vi "CRYStimulus Table Insert.vi"(9 "Insert":bool, 10 "Stimulus TableRef":refnum<vi>, 11 "Flatten Stimulus Setup String":string) -> (2 "Stimulus TableRef out":refnum<vi>)   [LabVIEW 2013]
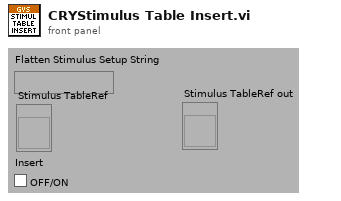
[diagram p1: front panel]
types:
  T1 = typedef "CRYfstepsw.ctl" = cluster{"Level(U)":dbl, "Start Freq(Hz)":dbl, "Stop Freq(Hz)":dbl, "ML val level name":string, "Use ML Val level?":bool, "ML axis":u8, "Steps (#)":i32, "Cycles/step(#)":u32, "Time/step (s)":dbl, "Step Resolution":u16, "unit":u16, "Start Freq Name":string, "Stop Freq Name":string, "Start Freq Axis":u8, "Stop Freq Axis":u8, "Start Freq Flag":string, "Stop Freq Flag":string, "Output Imp":dbl, "Nominal Imp":dbl, "V on DUT":bool}
  T2 = typedef "CRYflogsw.ctl" = cluster{"Level(U)":dbl, "Start Freq(Hz)":dbl, "Stop Freq(Hz)":dbl, "Sweep Rate(s/dec)":dbl, "Use ML Val level?":bool, "ML val level name":string, "ML axis":u8, "TSR params":cluster{"FSamp":dbl, "FStart":dbl, "FStop":dbl, "NOffset":dbl, "MStop":dbl, "MStart":dbl, "NHarm":dbl, "Tsamp":dbl, "Amplit":dbl}, "unit":u16, "Start Freq Name":string, "Stop Freq Name":string, "Start Freq Axis":u8, "Stop Freq Axis":u8, "Start Freq Flag":string, "Stop Freq Flag":string, "Output Imp":dbl, "Nominal Imp":dbl, "V on DUT":bool}
  T3 = typedef "CRYampsw.ctl" = cluster{"Freq(Hz)":dbl, "Steps (#)":i32, "Cycles(#)":u32, "Use ML Val freq?":bool, "ML val freq name":string, "ML axis":u8, "Start Ampl(U)":dbl, "Stop Ampl(U)":dbl, "unit":u16}
  T4 = typedef "CRYwavefile.ctl" = cluster{"Level(U)":dbl, "Wave Path":string, "ML axis":u8, "ML val level name":string, "Use ML Val level?":bool, "wave info":string, "wave time":string, "Peak value4":dbl, "RMS value4":dbl, "wave channel":u16, "unit":u16, "Output Imp":dbl, "Nominal Imp":dbl, "V on DUT":bool}
  T5 = typedef "CRYdcconn.ctl" = cluster{"dc ctrl":u16, "dcmax I":u16, "dc polar":u16, "dc ctrl":u16, "Steps (#)":i32, "Time/step (s)":dbl, "Start Ampl(U)":dbl, "Stop Ampl(U)":dbl, "Level(U)":dbl, "Step Size":dbl}
  T6 = typedef "CRYtwotone.ctl" = cluster{"Steps (#)":i32, "Tone Type":u8, "Freq2(Hz)":dbl, "Time/step (s)":dbl, "Cycles/step (#)":u32, "ML val level name":string, "Use ML Val level?":bool, "Level(U) 2":dbl, "Diff Freq(Hz)":dbl, "ML axis 2":u8, "Diff/Ratio":u8, "Level(U)":dbl, "Stop Freq(Hz)":dbl, "Ratio Val":dbl, "ML val level name 2":string, "Use ML Val level? 2":bool, "ML axis":u8, "Start Freq(Hz)":dbl, "Step Resolution":u16, "Ratio":u16, "TabCtrl6":enum32{"Master Tone", "Slave Tone"}, "unit 1":u16, "unit 2":u16, "Start Freq Name":string, "Stop Freq Name":string, "Start Freq Axis":u8, "Stop Freq Axis":u8, "Start Freq Flag":string, "Stop Freq Flag":string}
  T7 = typedef "CRYmltitone.ctl" = cluster{"Level(U)":dbl, "Min Freq(Hz)":dbl, "Max Freq(Hz)":dbl, "Duration(s)":dbl, "Freq Rounding":bool, "Rounding Val":dbl, "Profile":i32, "ML axis 2":u8, "ML val level name":string, "Use ML Val level?":bool, "ML axis":u8, "Step Resolution":u16, "unit":u16, "Start Freq Name":string, "Stop Freq Name":string, "Start Freq Axis":u8, "Stop Freq Axis":u8, "Start Freq Flag":string, "Stop Freq Flag":string, "Output Imp":dbl, "Nominal Imp":dbl, "V on DUT":bool}
  T8 = typedef "CRYnoise.ctl" = cluster{"Noise Type":u8, "Min Freq(Hz)":dbl, "Max Freq(Hz)":dbl, "Level(U)":dbl, "Duration(s)":dbl, "ML val level name":string, "Use ML Val level?":bool, "ML axis":u8, "unit":u16, "Start Freq Name":string, "Stop Freq Name":string, "Start Freq Axis":u8, "Stop Freq Axis":u8, "Start Freq Flag":string, "Stop Freq Flag":string, "Output Imp":dbl, "Nominal Imp":dbl, "V on DUT":bool}
  T9 = cluster{"fstepsw":T1, "flogsw":T2, "ampsw":T3, "wavefile":T4, "dcconn":T5, "twotone":T6, "mltitone":T7, "noise":T8, "sqwvsw":cluster{"Level(U)":dbl, "Duty Cycle":dbl, "ML val level name":string, "ML axis":u8, "Start Freq(Hz)":u32, "Stop Freq(Hz)":u32, "Use ML Val level?":bool, "Steps (#)":u32, "Cycles/step (#)":u32, "Time/step (s)":dbl, "Step Resolution":u16}, "tnbrst":cluster{"Level(U)":dbl, "ML val level name":string, "ML axis":u8, "Start Freq(Hz)":u32, "Use ML Val level?":bool, "Cycles/step (#)":u32, "Duration(s)":dbl}}
  T10 = cluster{"Data Type":string, "Version":u16, "Dimension":u8}
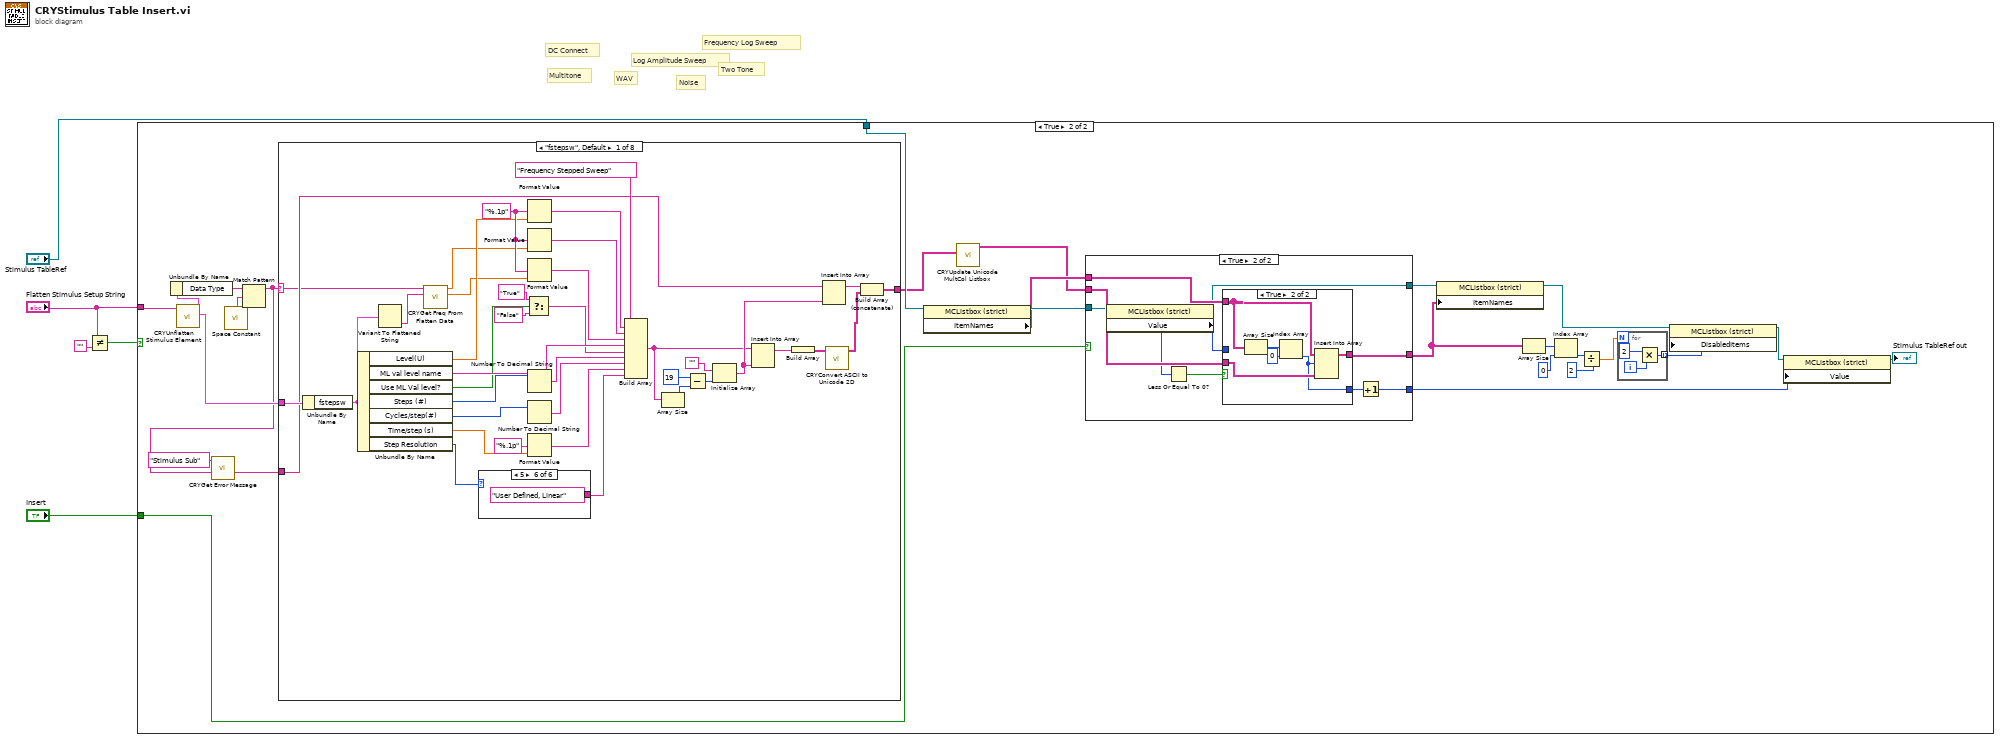
[diagram p0: block diagram]
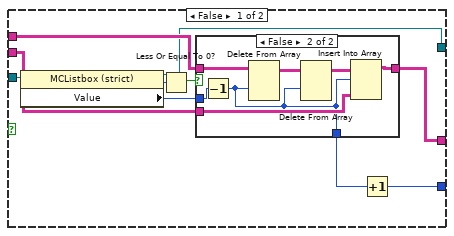
[diagram p3: hidden frame]
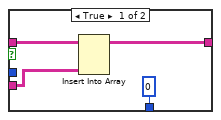
[diagram p4: hidden frame]
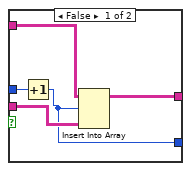
[diagram p5: hidden frame]
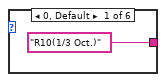
[diagram p6: hidden frame]
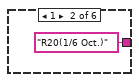
[diagram p7: hidden frame]
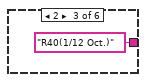
[diagram p8: hidden frame]
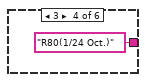
[diagram p9: hidden frame]
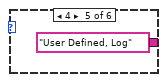
[diagram p10: hidden frame]
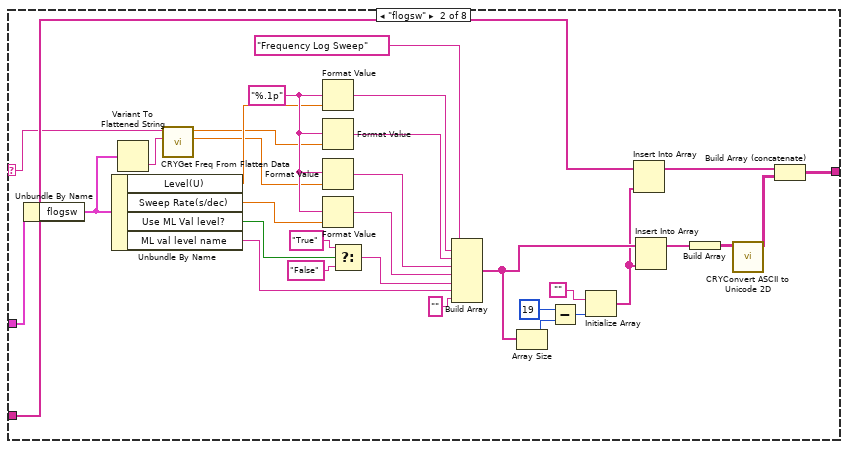
[diagram p11: hidden frame]
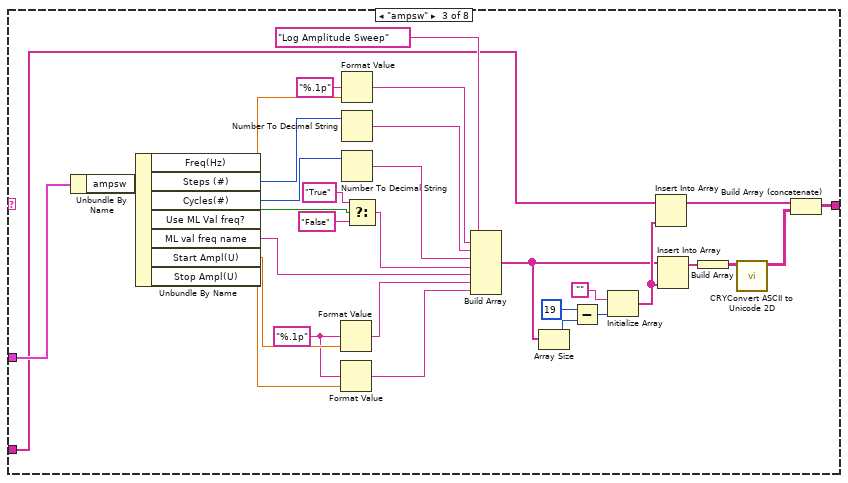
[diagram p12: hidden frame]
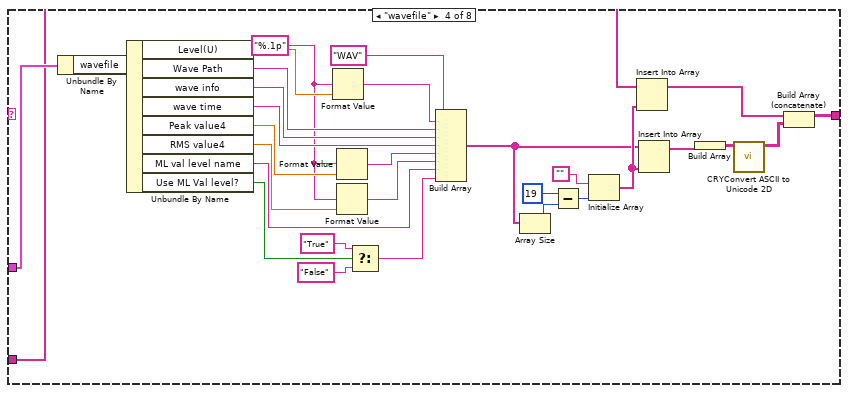
[diagram p13: hidden frame]
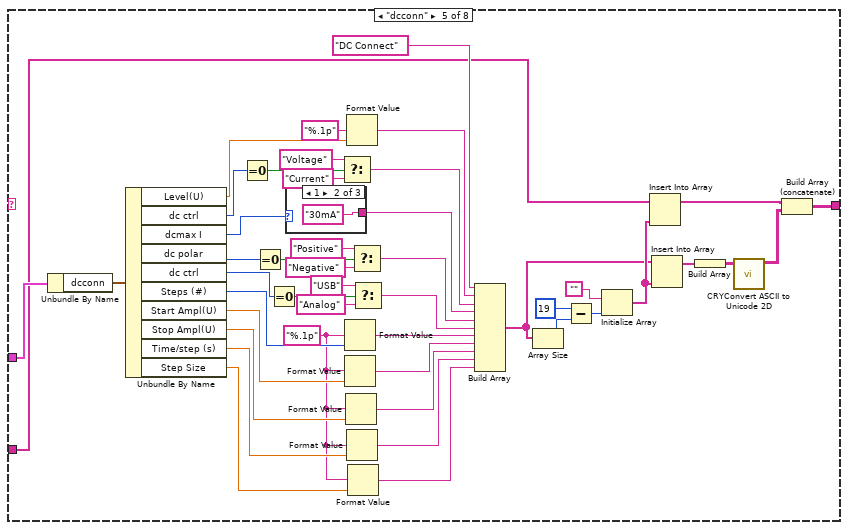
[diagram p14: hidden frame]
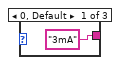
[diagram p15: hidden frame]
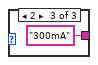
[diagram p16: hidden frame]
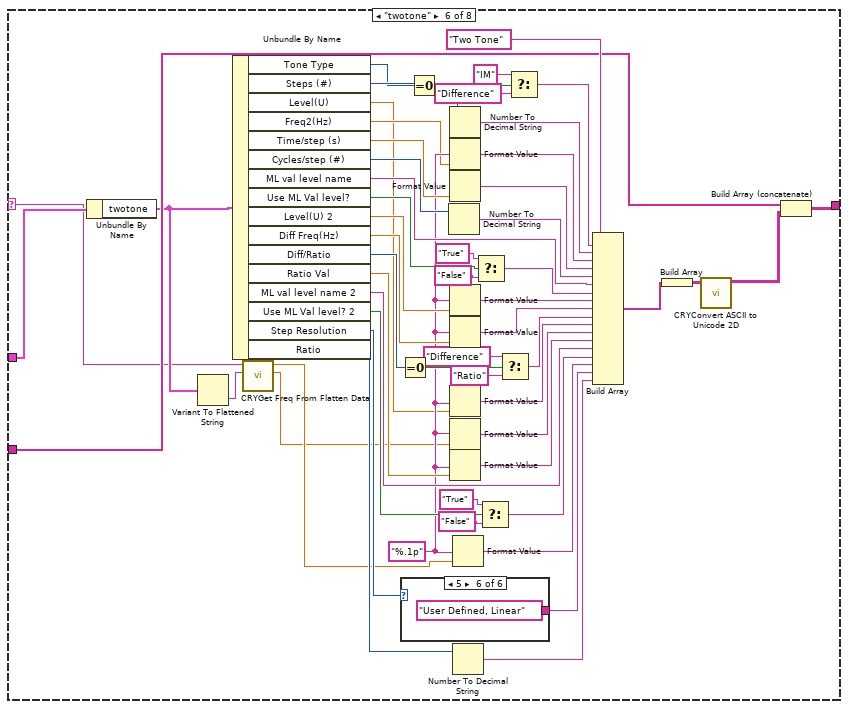
[diagram p17: hidden frame]
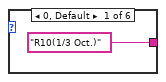
[diagram p18: hidden frame]
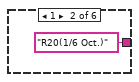
[diagram p19: hidden frame]
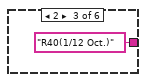
[diagram p20: hidden frame]
diagram:
  # "Multitone"
  # "Noise"
  # "Two Tone"
  # "DC Connect"
  # "WAV"
  # "Log Amplitude Sweep"
  # "Frequency Log Sweep"
  n1 = Not Equal?(x="Flatten Stimulus Setup String", y="") -> (x != y?=w4:bool)
  n2 = case shown="True" w4 {
    tunnel: "Flatten Stimulus Setup String" -> [_ w6]
    tunnel: "Stimulus TableRef" -> [_ w20]
    tunnel: "Insert" -> [_ w21]
    frame False {
    }
    frame True {
      n3 = call "CRYUnflatten Stimulus Element.vi"("Unflatten Stimulus Element setup"=w6) -> ("Stimulus Default"=w30:T9, "Header of common"=w31:T10)  [unwired: 1 in, 8 out]
      n4 = Unbundle By Name(w31) -> ("Data Type"=w29:string)
      n5 = call <vilib>:"Space Constant.vi"() -> ("String"=w28:string)
      n6 = Match Pattern(string=w29, regular expression=w28) -> (before substring=w7:string)  [unwired: 4 out]
      n7 = call "CRYGet Error Message.vi"("String In"=w7, "Kind"="Stimulus Sub") -> ("Unicode Message Sub"=w15:string[])  [unwired: 4 in, 5 out]
      n8 = case shown="\"fstepsw\", Default" w7 {
        selector: w7 -> [w77 w121 _ _ _ w264 w325 w361]
        tunnel: w30 -> [w112 w150 w176 w210 w253 w300 w353 w390]
        tunnel: [w102 w142 w171 w209 w252 w299 w352 w391] -> w12
        tunnel: w15 -> [w86 w130 w155 w187 w217 w270 w334 w369]
        frame "fstepsw", Default {
          w92 = "%.1p" ("format string")
          n9 = Unbundle By Name(w112) -> ("fstepsw"=w79:T1)
          n10 = Unbundle By Name(w79) -> ("Level(U)"=w80:dbl, "ML val level name"=w106:string, "Use ML Val level?"=w98:bool, "Steps (#)"=w111:i32, "Cycles/step(#)"=w110:u32, "Time/step (s)"=w94:dbl, "Step Resolution"=w100:u16)
          n11 = Variant To Flattened String(Variant=w79) -> (data string=w78:string)  [unwired: 1 out]
          n12 = call "CRYGet Freq From Flatten Data.vi"("Flattened Element Data"=w78, "Stimulus Type"=w77) -> ("Stop Freq(Hz)"=w75:dbl, "Start Freq(Hz)"=w76:dbl)  [unwired: 8 in]
          n13 = case shown="5" w100 {
            tunnel: ["R10(1/3 Oct.)" "R20(1/6 Oct.)" "R40(1/12 Oct.)" "R80(1/24 Oct.)" "User Defined, Log" "User Defined, Linear"] -> w99
            frame 0, Default {
            }
            frame 1 {
            }
            frame 2 {
            }
            frame 3 {
            }
            frame 4 {
            }
            frame 5 {
            }
          }
          n14 = Select(t="True", s=w98, f="False") -> (s? t:f=w95:string)
          n15 = Format Value(format string=w92, value (0)=w80) -> (output string=w109:string)  [unwired: 1 in]
          n16 = Format Value(format string=w92, value (0)=w76) -> (output string=w108:string)  [unwired: 1 in]
          n17 = Format Value(format string=w92, value (0)=w75) -> (output string=w107:string)  [unwired: 1 in]
          n18 = Number To Decimal String(number=w111) -> (decimal integer string=w105:string)  [unwired: 1 out]
          n19 = Number To Decimal String(number=w110) -> (decimal integer string=w104:string)  [unwired: 1 out]
          n20 = Format Value(format string="%.1p", value (0)=w94) -> (output string=w103:string)  [unwired: 1 in]
          n21 = Build Array("Frequency Stepped Sweep" ("element"), w109, w108, w107, w106, w95, w105, w104, w103, w99) -> (w85:string[])
          n22 = Array Size(array=w85) -> (size(s)=w91:i32)
          n23 = Subtract(x=19, y=w91) -> (x-y=w89:i32)
          n24 = Initialize Array("", w89) -> (w87:string[])
          n25 = Insert Into Array(array=w85, new element=w87) -> (w83:string[])  [unwired: 1 in]
          n26 = Build Array(w83) -> (w82:string[][])
          n27 = Insert Into Array(array=w86, new element=w87) -> (w84:string[])  [unwired: 1 in]
          n28 = call "CRYConvert ASCII to Unicode 2D.vi"("ASCII"=w82) -> ("Unicode"=w81:string[][])  [unwired: 10 in]
          n29 = Build Array (concatenate)(w84, w81) -> (w102:string[][])
        }
        frame "flogsw" {
          w136 = "%.1p" ("format string")
          n30 = Unbundle By Name(w150) -> ("flogsw"=w122:T2)
          n31 = Unbundle By Name(w122) -> ("Level(U)"=w124:dbl, "Sweep Rate(s/dec)"=w137:dbl, "Use ML Val level?"=w141:bool, "ML val level name"=w144:string)
          n32 = Variant To Flattened String(Variant=w122) -> (data string=w123:string)  [unwired: 1 out]
          n33 = call "CRYGet Freq From Flatten Data.vi"("Flattened Element Data"=w123, "Stimulus Type"=w121) -> ("Stop Freq(Hz)"=w119:dbl, "Start Freq(Hz)"=w120:dbl)  [unwired: 8 in]
          n34 = Format Value(format string=w136, value (0)=w124) -> (output string=w149:string)  [unwired: 1 in]
          n35 = Format Value(format string=w136, value (0)=w120) -> (output string=w148:string)  [unwired: 1 in]
          n36 = Format Value(format string=w136, value (0)=w119) -> (output string=w147:string)  [unwired: 1 in]
          n37 = Format Value(format string=w136, value (0)=w137) -> (output string=w146:string)  [unwired: 1 in]
          n38 = Select(t="True", s=w141, f="False") -> (s? t:f=w138:string)
          n39 = Build Array("Frequency Log Sweep" ("element"), w149, w148, w147, w146, w138, w144, "" ("element")) -> (w131:string[])
          n40 = Array Size(array=w131) -> (size(s)=w135:i32)
          n41 = Subtract(x=19, y=w135) -> (x-y=w133:i32)
          n42 = Initialize Array("", w133) -> (w129:string[])
          n43 = Insert Into Array(array=w130, new element=w129) -> (w128:string[])  [unwired: 1 in]
          n44 = Insert Into Array(array=w131, new element=w129) -> (w127:string[])  [unwired: 1 in]
          n45 = Build Array(w127) -> (w126:string[][])
          n46 = call "CRYConvert ASCII to Unicode 2D.vi"("ASCII"=w126) -> ("Unicode"=w125:string[][])  [unwired: 10 in]
          n47 = Build Array (concatenate)(w128, w125) -> (w142:string[][])
        }
        frame "ampsw" {
          w162 = "%.1p" ("format string")
          n48 = Unbundle By Name(w176) -> ("ampsw"=w182:T3)
          n49 = Unbundle By Name(w182) -> ("Freq(Hz)"=w166:dbl, "Steps (#)"=w175:i32, "Cycles(#)"=w174:u32, "Use ML Val freq?"=w170:bool, "ML val freq name"=w173:string, "Start Ampl(U)"=w164:dbl, "Stop Ampl(U)"=w163:dbl)
          n50 = Format Value(format string=w162, value (0)=w164) -> (output string=w178:string)  [unwired: 1 in]
          n51 = Format Value(format string=w162, value (0)=w163) -> (output string=w172:string)  [unwired: 1 in]
          n52 = Format Value(format string="%.1p", value (0)=w166) -> (output string=w181:string)  [unwired: 1 in]
          n53 = Number To Decimal String(number=w175) -> (decimal integer string=w180:string)  [unwired: 1 out]
          n54 = Number To Decimal String(number=w174) -> (decimal integer string=w179:string)  [unwired: 1 out]
          n55 = Select(t="True", s=w170, f="False") -> (s? t:f=w168:string)
          n56 = Build Array("Log Amplitude Sweep" ("element"), w181, w180, w179, w168, w173, w178, w172) -> (w156:string[])
          n57 = Array Size(array=w156) -> (size(s)=w161:i32)
          n58 = Subtract(x=19, y=w161) -> (x-y=w159:i32)
          n59 = Initialize Array("", w159) -> (w157:string[])
          n60 = Insert Into Array(array=w155, new element=w157) -> (w154:string[])  [unwired: 1 in]
          n61 = Insert Into Array(array=w156, new element=w157) -> (w153:string[])  [unwired: 1 in]
          n62 = Build Array(w153) -> (w152:string[][])
          n63 = call "CRYConvert ASCII to Unicode 2D.vi"("ASCII"=w152) -> ("Unicode"=w151:string[][])  [unwired: 10 in]
          n64 = Build Array (concatenate)(w154, w151) -> (w171:string[][])
        }
        frame "wavefile" {
          w194 = "%.1p" ("format string")
          n65 = Unbundle By Name(w210) -> ("wavefile"=w212:T4)
          n66 = Unbundle By Name(w212) -> ("Level(U)"=w197:dbl, "Wave Path"=w208:string, "wave info"=w206:string, "wave time"=w205:string, "Peak value4"=w196:dbl, "RMS value4"=w195:dbl, "ML val level name"=w202:string, "Use ML Val level?"=w201:bool)
          n67 = Format Value(format string=w194, value (0)=w197) -> (output string=w207:string)  [unwired: 1 in]
          n68 = Format Value(format string=w194, value (0)=w196) -> (output string=w204:string)  [unwired: 1 in]
          n69 = Format Value(format string=w194, value (0)=w195) -> (output string=w203:string)  [unwired: 1 in]
          n70 = Select(t="True", s=w201, f="False") -> (s? t:f=w198:string)
          n71 = Build Array("WAV" ("element"), w207, w208, w206, w205, w204, w203, w202, w198) -> (w188:string[])
          n72 = Array Size(array=w188) -> (size(s)=w193:i32)
          n73 = Subtract(x=19, y=w193) -> (x-y=w191:i32)
          n74 = Initialize Array("", w191) -> (w189:string[])
          n75 = Insert Into Array(array=w187, new element=w189) -> (w186:string[])  [unwired: 1 in]
          n76 = Insert Into Array(array=w188, new element=w189) -> (w185:string[])  [unwired: 1 in]
          n77 = Build Array(w185) -> (w184:string[][])
          n78 = call "CRYConvert ASCII to Unicode 2D.vi"("ASCII"=w184) -> ("Unicode"=w183:string[][])  [unwired: 10 in]
          n79 = Build Array (concatenate)(w186, w183) -> (w209:string[][])
        }
        frame "dcconn" {
          w224 = "%.1p" ("format string")
          n80 = Unbundle By Name(w253) -> ("dcconn"=w258:T5)
          n81 = Unbundle By Name(w258) -> ("Level(U)"=w231:dbl, "dc ctrl"=w249:u16, "dcmax I"=w244:u16, "dc polar"=w240:u16, "dc ctrl"=w236:u16, "Steps (#)"=w229:i32, "Start Ampl(U)"=w228:dbl, "Stop Ampl(U)"=w227:dbl, "Time/step (s)"=w226:dbl, "Step Size"=w225:dbl)
          n82 = Equal To 0?(x=w249) -> (x = 0?=w248:bool)
          n83 = Equal To 0?(x=w240) -> (x = 0?=w241:bool)
          n84 = Equal To 0?(x=w236) -> (x = 0?=w238:bool)
          n85 = case shown="1" w244 {
            tunnel: ["3mA" ("element") "30mA" ("element") "300mA" ("element")] -> w243
            frame 0, Default {
            }
            frame 1 {
            }
            frame 2 {
            }
          }
          n86 = Select(t="Voltage" ("element"), s=w248, f="Current" ("element")) -> (s? t:f=w245:string)
          n87 = Format Value(format string=w224, value (0)=w229) -> (output string=w251:string)  [unwired: 1 in]
          n88 = Format Value(format string=w224, value (0)=w228) -> (output string=w254:string)  [unwired: 1 in]
          n89 = Format Value(format string=w224, value (0)=w227) -> (output string=w257:string)  [unwired: 1 in]
          n90 = Format Value(format string="%.1p", value (0)=w231) -> (output string=w250:string)  [unwired: 1 in]
          n91 = Format Value(format string=w224, value (0)=w226) -> (output string=w255:string)  [unwired: 1 in]
          n92 = Format Value(format string=w224, value (0)=w225) -> (output string=w232:string)  [unwired: 1 in]
          n93 = Select(t="Positive" ("element"), s=w241, f="Negative" ("element")) -> (s? t:f=w239:string)
          n94 = Select(t="USB" ("element"), s=w238, f="Analog" ("element")) -> (s? t:f=w233:string)
          n95 = Build Array("DC Connect" ("element"), w250, w245, w243, w239, w233, w251, w254, w257, w255, w232) -> (w218:string[])
          n96 = Array Size(array=w218) -> (size(s)=w223:i32)
          n97 = Subtract(x=19, y=w223) -> (x-y=w221:i32)
          n98 = Initialize Array("", w221) -> (w219:string[])
          n99 = Insert Into Array(array=w217, new element=w219) -> (w216:string[])  [unwired: 1 in]
          n100 = Insert Into Array(array=w218, new element=w219) -> (w215:string[])  [unwired: 1 in]
          n101 = Build Array(w215) -> (w214:string[][])
          n102 = call "CRYConvert ASCII to Unicode 2D.vi"("ASCII"=w214) -> ("Unicode"=w213:string[][])  [unwired: 10 in]
          n103 = Build Array (concatenate)(w216, w213) -> (w252:string[][])
        }
        frame "twotone" {
          w273 = "%.1p" ("format string")
          n104 = Unbundle By Name(w300) -> ("twotone"=w265:T6)
          n105 = Variant To Flattened String(Variant=w265) -> (data string=w266:string)  [unwired: 1 out]
          n106 = Unbundle By Name(w265) -> ("Tone Type"=w296:u8, "Steps (#)"=w305:i32, "Level(U)"=w271:dbl, "Freq2(Hz)"=w272:dbl, "Time/step (s)"=w276:dbl, "Cycles/step (#)"=w304:u32, "ML val level name"=w303:string, "Use ML Val level?"=w292:bool, "Level(U) 2"=w275:dbl, "Diff Freq(Hz)"=w277:dbl, "Diff/Ratio"=w285:u8, "Ratio Val"=w274:dbl, "ML val level name 2"=w302:string, "Use ML Val level? 2"=w281:bool, "Step Resolution"=w279:u16, "Ratio"=w301:u16)
          n107 = call "CRYGet Freq From Flatten Data.vi"("Flattened Element Data"=w266, "Stimulus Type"=w264) -> ("Stop Freq(Hz)"=w262:dbl, "Start Freq(Hz)"=w263:dbl)  [unwired: 8 in]
          n108 = Equal To 0?(x=w285) -> (x = 0?=w286:bool)
          n109 = case shown="5" w279 {
            tunnel: ["R10(1/3 Oct.)" "R20(1/6 Oct.)" "R40(1/12 Oct.)" "R80(1/24 Oct.)" "User Defined, Log" "User Defined, Linear"] -> w278
            frame 0, Default {
            }
            frame 1 {
            }
            frame 2 {
            }
            frame 3 {
            }
            frame 4 {
            }
            frame 5 {
            }
          }
          n110 = Equal To 0?(x=w296) -> (x = 0?=w297:bool)
          n111 = Number To Decimal String(number=w304) -> (decimal integer string=w312:string)  [unwired: 1 out]
          n112 = Number To Decimal String(number=w305) -> (decimal integer string=w316:string)  [unwired: 1 out]
          n113 = Format Value(format string=w273, value (0)=w272) -> (output string=w315:string)  [unwired: 1 in]
          n114 = Format Value(value (0)=w276) -> (output string=w313:string)  [unwired: 1 in, 1 out]
          n115 = Format Value(format string=w273, value (0)=w275) -> (output string=w311:string)  [unwired: 1 in]
          n116 = Format Value(format string=w273, value (0)=w277) -> (output string=w310:string)  [unwired: 1 in]
          n117 = Format Value(format string=w273, value (0)=w271) -> (output string=w309:string)  [unwired: 1 in]
          n118 = Format Value(format string=w273, value (0)=w262) -> (output string=w308:string)  [unwired: 1 in]
          n119 = Format Value(format string=w273, value (0)=w274) -> (output string=w307:string)  [unwired: 1 in]
          n120 = Format Value(format string=w273, value (0)=w263) -> (output string=w306:string)  [unwired: 1 in]
          n121 = Number To Decimal String(number=w301) -> (decimal integer string=w298:string)  [unwired: 1 out]
          n122 = Select(t="True", s=w292, f="False") -> (s? t:f=w289:string)
          n123 = Select(t="True", s=w281, f="False") -> (s? t:f=w280:string)
          n124 = Select(t="Difference" ("element"), s=w286, f="Ratio" ("element")) -> (s? t:f=w284:string)
          n125 = Select(t="IM" ("element"), s=w297, f="Difference" ("element")) -> (s? t:f=w293:string)
          n126 = Build Array("Two Tone" ("element"), w293, w316, w315, w313, w312, w303, w289, w311, w310, w284, w309, w308, w307, w302, w280, w306, w278, w298) -> (w269:string[])
          n127 = Build Array(w269) -> (w268:string[][])
          n128 = call "CRYConvert ASCII to Unicode 2D.vi"("ASCII"=w268) -> ("Unicode"=w267:string[][])  [unwired: 10 in]
          n129 = Build Array (concatenate)(w270, w267) -> (w299:string[][])
        }
        frame "noise" {
          w340 = "%.1p" ("format string")
          n130 = Unbundle By Name(w353) -> ("noise"=w326:T8)
          n131 = Unbundle By Name(w326) -> ("Noise Type"=w328:u8, "Level(U)"=w342:dbl, "Duration(s)"=w341:dbl, "ML val level name"=w351:string, "Use ML Val level?"=w344:bool)
          n132 = Variant To Flattened String(Variant=w326) -> (data string=w327:string)  [unwired: 1 out]
          n133 = call "CRYGet Freq From Flatten Data.vi"("Flattened Element Data"=w327, "Stimulus Type"=w325) -> ("Stop Freq(Hz)"=w324:dbl, "Start Freq(Hz)"=w323:dbl)  [unwired: 8 in]
          n134 = Equal To 0?(x=w328) -> (x = 0?=w350:bool)
          n135 = Format Value(format string=w340, value (0)=w341) -> (output string=w354:string)  [unwired: 1 in]
          n136 = Format Value(format string=w340, value (0)=w323) -> (output string=w358:string)  [unwired: 1 in]
          n137 = Format Value(format string=w340, value (0)=w324) -> (output string=w357:string)  [unwired: 1 in]
          n138 = Format Value(format string=w340, value (0)=w342) -> (output string=w355:string)  [unwired: 1 in]
          n139 = Select(t="Pink" ("element"), s=w350, f="White" ("element")) -> (s? t:f=w347:string)
          n140 = Select(t="True", s=w344, f="False") -> (s? t:f=w343:string)
          n141 = Build Array("Noise" ("element"), w347, w358, w357, w355, w354, w351, w343) -> (w333:string[])
          n142 = Array Size(array=w333) -> (size(s)=w339:i32)
          n143 = Subtract(x=19, y=w339) -> (x-y=w337:i32)
          n144 = Initialize Array("", w337) -> (w335:string[])
          n145 = Insert Into Array(array=w334, new element=w335) -> (w332:string[])  [unwired: 1 in]
          n146 = Insert Into Array(array=w333, new element=w335) -> (w331:string[])  [unwired: 1 in]
          n147 = Build Array(w331) -> (w330:string[][])
          n148 = call "CRYConvert ASCII to Unicode 2D.vi"("ASCII"=w330) -> ("Unicode"=w329:string[][])  [unwired: 10 in]
          n149 = Build Array (concatenate)(w332, w329) -> (w352:string[][])
        }
        frame "mltitone" {
          w376 = "%.1p" ("format string")
          n150 = Unbundle By Name(w390) -> ("mltitone"=w362:T7)
          n151 = Unbundle By Name(w362) -> ("Level(U)"=w364:dbl, "Duration(s)"=w377:dbl, "Freq Rounding"=w384:bool, "Rounding Val"=w378:dbl, "Profile"=w389:i32, "ML val level name"=w388:string, "Use ML Val level?"=w380:bool, "Step Resolution"=w387:u16)
          n152 = Variant To Flattened String(Variant=w362) -> (data string=w363:string)  [unwired: 1 out]
          n153 = call "CRYGet Freq From Flatten Data.vi"("Flattened Element Data"=w363, "Stimulus Type"=w361) -> ("Stop Freq(Hz)"=w359:dbl, "Start Freq(Hz)"=w360:dbl)  [unwired: 8 in]
          n154 = Format Value(format string=w376, value (0)=w364) -> (output string=w399:string)  [unwired: 1 in]
          n155 = Format Value(format string=w376, value (0)=w360) -> (output string=w398:string)  [unwired: 1 in]
          n156 = Format Value(format string=w376, value (0)=w359) -> (output string=w397:string)  [unwired: 1 in]
          n157 = Format Value(format string=w376, value (0)=w377) -> (output string=w395:string)  [unwired: 1 in]
          n158 = Format Value(format string=w376, value (0)=w378) -> (output string=w394:string)  [unwired: 1 in]
          n159 = Number To Decimal String(number=w389) -> (decimal integer string=w393:string)  [unwired: 1 out]
          n160 = Number To Decimal String(number=w387) -> (decimal integer string=w392:string)  [unwired: 1 out]
          n161 = Select(t="True", s=w384, f="False") -> (s? t:f=w383:string)
          n162 = Select(t="True", s=w380, f="False") -> (s? t:f=w379:string)
          n163 = Build Array("Multitone" ("element"), w399, w398, w397, w395, w383, w394, w393, w388, w379, w392) -> (w370:string[])
          n164 = Array Size(array=w370) -> (size(s)=w375:i32)
          n165 = Subtract(x=19, y=w375) -> (x-y=w373:i32)
          n166 = Initialize Array("", w373) -> (w371:string[])
          n167 = Insert Into Array(array=w369, new element=w371) -> (w368:string[])  [unwired: 1 in]
          n168 = Insert Into Array(array=w370, new element=w371) -> (w367:string[])  [unwired: 1 in]
          n169 = Build Array(w367) -> (w366:string[][])
          n170 = call "CRYConvert ASCII to Unicode 2D.vi"("ASCII"=w366) -> ("Unicode"=w365:string[][])  [unwired: 10 in]
          n171 = Build Array (concatenate)(w368, w365) -> (w391:string[][])
        }
      }
      n172 = property on="Property Node" class="MCListbox (strict)"(reference=w20) -> (reference out=w14:refnum<vi>, "ItemNames"=w13:string[][])  [unwired: 1 in, 1 out]
      n173 = call "CRYUpdate Unicode MultCol Listbox.vi"("Data[]"=w12) -> ("Data[] Out"=w11:string[][])  [unwired: 8 in]
      n174 = case shown="True" w21 {
        tunnel: w11 -> [w38 w60]
        tunnel: w14 -> [w40 w59]
        tunnel: [w34 w52] -> w19
        tunnel: [w37 w56] -> w8
        tunnel: [w36 w53] -> w10
        tunnel: w13 -> [w39 w54]
        frame False {
          n175 = property on="Property Node" class="MCListbox (strict)"(reference=w40) -> (reference out=w36:refnum<vi>, "Value"=w33:i32)  [unwired: 1 in, 1 out]
          n176 = Less Or Equal To 0?(x=w33) -> (x <= 0?=w32:bool)
          n177 = case shown="False" w32 {
            tunnel: w33 -> [_ w51]
            tunnel: w39 -> [w43 w50]
            tunnel: w38 -> [w42 w47]
            tunnel: [w41 w46] -> w37
            tunnel: [0 w45] -> w35
            frame True {
              n178 = Insert Into Array(array=w43, new element=w42) -> (w41:string[][])  [unwired: 2 in]
            }
            frame False {
              n179 = Decrement(x=w51) -> (x-1=w45:i32)
              n180 = Delete From Array(array=w50, index (row)=w45) -> (array with subset deleted=w49:string[][])  [unwired: 2 in, 1 out]
              n181 = Delete From Array(array=w49, index (row)=w45) -> (array with subset deleted=w48:string[][])  [unwired: 2 in, 1 out]
              n182 = Insert Into Array(array=w48, index (row)=w45, new element=w47) -> (w46:string[][])  [unwired: 1 in]
            }
          }
          n183 = Increment(x=w35) -> (x+1=w34:i32)
        }
        frame True {
          n184 = property on="Property Node" class="MCListbox (strict)"(reference=w59) -> (reference out=w53:refnum<vi>, "Value"=w55:i32)  [unwired: 1 in, 1 out]
          n185 = Less Or Equal To 0?(x=w55) -> (x <= 0?=w57:bool)
          n186 = case shown="True" w57 {
            tunnel: w54 -> [w64 w69]
            tunnel: w60 -> [w65 w68]
            tunnel: w55 -> [w62 _]
            tunnel: [w63 w67] -> w56
            tunnel: [w61 w66] -> w58
            frame False {
              n187 = Increment(x=w62) -> (x+1=w61:i32)
              n188 = Insert Into Array(array=w64, index (row)=w61, new element=w65) -> (w63:string[][])  [unwired: 1 in]
            }
            frame True {
              n189 = Array Size(array=w69) -> (size(s)=w71:i32[])
              n190 = Index Array(array=w71, index=0) -> (element=w66:i32)
              n191 = Insert Into Array(array=w69, index (row)=w66, new element=w68) -> (w67:string[][])  [unwired: 1 in]
            }
          }
          n192 = Increment(x=w58) -> (x+1=w52:i32)
        }
      }
      n193 = property class="MCListbox (strict)"(reference=w10, "ItemNames"=w8) -> (reference out=w9:refnum<vi>)  [unwired: 1 in, 1 out]
      n194 = Array Size(array=w8) -> (size(s)=w27:i32[])
      n195 = Index Array(array=w27, index=0) -> (element=w25:i32)
      n196 = Divide(x=w25, y=2) -> (x/y=w23:dbl)
      n197 = for {
        N: w23 -> [_]
        tunnel: [w72] -> w22 mode=indexing
        i -> [w74]
        n198 = Multiply(x=2, y=w74) -> (x*y=w72:i32)
      }
      n199 = property on="Property Node" class="MCListbox (strict)"(reference=w9, "DisabledItems"=w22) -> (reference out=w18:refnum<vi>)  [unwired: 1 in, 1 out]
      n200 = property on="Property Node" class="MCListbox (strict)"(reference=w18, "Value"=w19) -> (reference out=→"Stimulus TableRef out":refnum<vi>)  [unwired: 1 in, 1 out]
    }
  }
